vi "Setup.vi"(8 "Error In":errorcluster) -> (0 "Error Out":errorcluster, 3 "File Info":refnum<class "File Info.lvclass">)   [LabVIEW 2018, in "Tests.lvlib" / "File Info.lvlib"]
uses:
  File Info.lvlib
  src/Toolkit/File Info/File Info.lvclass
  src/Toolkit/File Info/Support/Create from SSH.vi
  src/Toolkit/SSH/SSH.lvclass
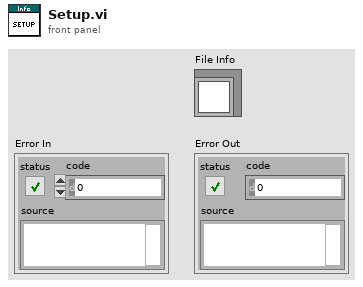
[diagram p1: front panel]
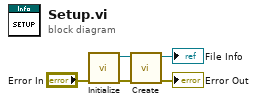
[diagram p0: block diagram]
diagram:
  n1 = call "Initialize.vi"("Error In"="Error In") -> ("Error Out"=w3:errorcluster, "SSH"=w4:refnum<class "SSH.lvclass">)  [unwired: 9 in]
  n2 = call-poly "Create.vi"("Error In"=w3, "SSH"=w4) -> ("Error Out"=→"Error Out":errorcluster, "File Info"=→"File Info":refnum<class "File Info.lvclass">)  [unwired: 8 in]
